vi "Deflection correction.vi"(8 "fitted piezo":dbl[](array[numeric]), 9 "psd":dbl[](array[numeric]), 10 "spring constant [N/m]":dbl, 11 "RT DEFLECTION CORRECTION":bool) -> (3 "Array":cluster{dbl[], dbl[]}[](array[cluster]))   [LabVIEW 2013]
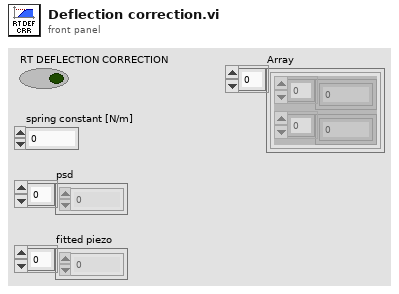
[diagram p1: front panel]
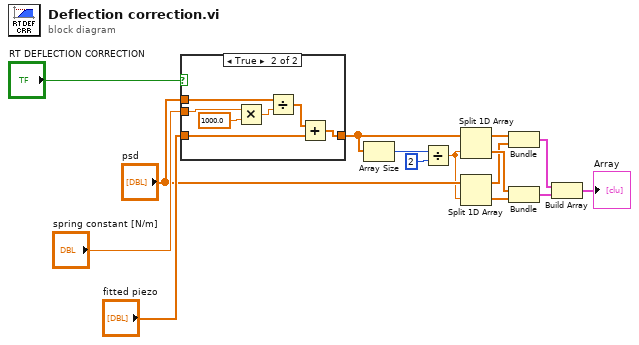
[diagram p0: block diagram]
diagram:
  n1 = case shown="True" "RT DEFLECTION CORRECTION" {
    tunnel: "fitted piezo" -> [w16 w22]
    tunnel: [w16 w21] -> w3
    tunnel: "spring constant [N/m]" -> [_ w18]
    tunnel: "psd" -> [_ w17]
    frame False {
    }
    frame True {
      n2 = Multiply(x=w18, y=1000.0) -> (x*y=w19:dbl)
      n3 = Divide(x=w17, y=w19) -> (x/y=w23:dbl[])
      n4 = Add(x=w23, y=w22) -> (x+y=w21:dbl[])
    }
  }
  n5 = Array Size(array=w3) -> (size(s)=w4:i32)
  n6 = Divide(x=w4, y=2) -> (x/y=w6:dbl)
  n7 = Split 1D Array(array=w3, index=w6) -> (first subarray=w7:dbl[], second subarray=w9:dbl[])
  n8 = Split 1D Array(array="psd", index=w6) -> (first subarray=w8:dbl[], second subarray=w10:dbl[])
  n9 = Bundle(w7, w8) -> (w2:cluster{dbl[], dbl[]})  [unwired: 1 in]
  n10 = Bundle(w9, w10) -> (w1:cluster{dbl[], dbl[]})  [unwired: 1 in]
  n11 = Build Array(w2, w1) -> (→"Array":cluster{dbl[], dbl[]}[])
